vi "strip all highlighting.vi"(0 "input string":string) -> (3 "Selection":bool, 4 "stripped output":string, 6 "highlighted strings":string[](array[string]), 8 "highlighted lines":i32[](array[numeric]), 10 "Selection cluster":cluster{i32, i32, "selected string":string}, 15 "error out":errorcluster)   [LabVIEW 2018]
uses:
  <userlib>/_OpenG.lib/array/array.llb/Search 1D Array (Boolean)__ogtk.vi
panel:
  out "Highlighting":bool
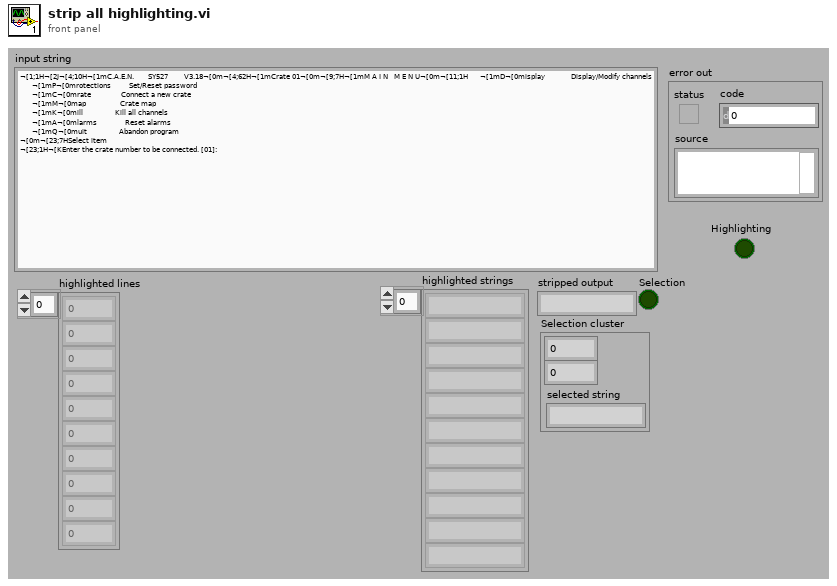
[diagram p1: front panel]
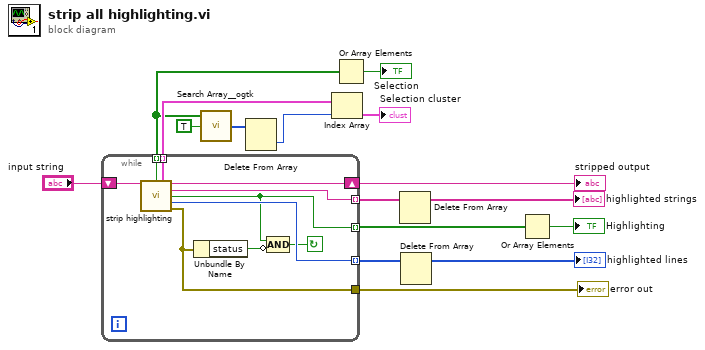
[diagram p0: block diagram]
diagram:
  n1 = while {
    shift-right: [w25] -> w12
    shift-left: "input string" -> [w26]
    tunnel: [w24] -> w11 mode=indexing
    tunnel: [w20] -> w15 mode=indexing
    tunnel: [w23] -> w9 mode=indexing
    tunnel: [w22] -> w13
    tunnel: [w18] -> w7 mode=indexing
    tunnel: [w17] -> w2 mode=indexing
    stop <- w19 continue-if-true
    n2 = call "strip highlighting.vi"("input string"=w26) -> ("Selection"=w17:bool, "Selection cluster"=w18:cluster{i32, i32, "selected string":string}, "output string"=w25:string, "Highlighted string"=w24:string, "Highlighting"=w20:bool, "Line #"=w23:i32, "error out"=w22:errorcluster)  [unwired: 8 in]
    n3 = Unbundle By Name(w22) -> ("status"=w21:bool)
    n4 = Compound Arithmetic op=AND(w20, invert w21) -> (w19:bool)
  }
  "error out" <- w13
  "stripped output" <- w12
  n5 = call-poly <userlib>:"Search Array__ogtk.vi"("Array"=w2, "Element Data"=TRUE ("element")) -> ("Indices of Elements"=w4:i32[])  [unwired: 7 in]
  n6 = Delete From Array(array=w4) -> (deleted portion=w3:i32)  [unwired: 2 in, 1 out]
  n7 = Index Array(array=w7, index=w3) -> (element=→"Selection cluster":cluster{i32, i32, "selected string":string})
  n8 = Or Array Elements(Boolean array=w2) -> (logical OR=→"Selection":bool)
  n9 = Delete From Array(array=w11) -> (array with subset deleted=→"highlighted strings":string[])  [unwired: 2 in, 1 out]
  n10 = Delete From Array(array=w9) -> (array with subset deleted=→"highlighted lines":i32[])  [unwired: 2 in, 1 out]
  n11 = Or Array Elements(Boolean array=w15) -> (logical OR=→"Highlighting":bool)
